vi "subVI_load_cell_KA.vi"(9 "offset":dbl, 10 "scale":dbl=1.0, 11 "DATA ARRAY IN":bool[](array[boolean])) -> (3 "LOAD OUT":dbl)   [LabVIEW 2018]
panel:
  out "decimal number":i32
  out "32 bit Zero padded array":bool[](array[boolean])
  out "24 bit Data array":bool[](array[boolean])
  # "This Sub-VI takes the Boolean Array from the Load Cell Amplifier\nand converts it into a load using the scale and offset from calibration"
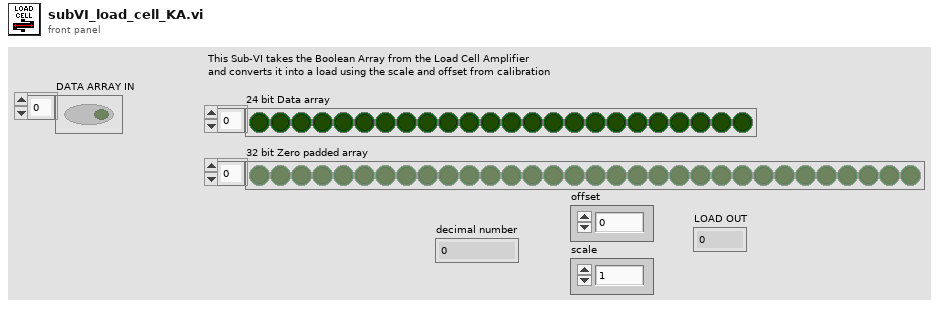
[diagram p1: front panel]
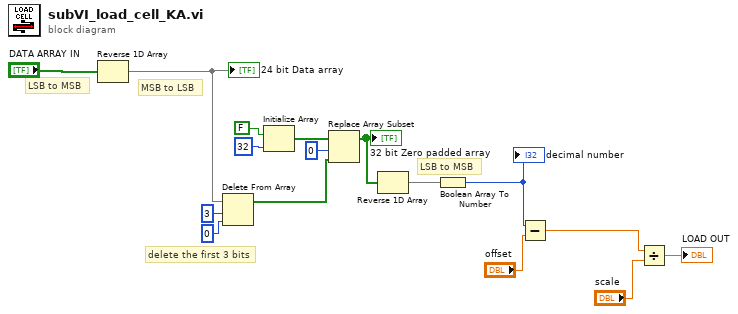
[diagram p0: block diagram]
diagram:
  # "LSB to MSB"
  # "delete the first 3 bits"
  # "LSB to MSB"
  # "MSB to LSB"
  n1 = Reverse 1D Array(array="DATA ARRAY IN") -> (reversed array=w6:bool[])
  "24 bit Data array" <- w6
  n2 = Delete From Array(array=w6, length=3, index=0) -> (array with subset deleted=w3:bool[])  [unwired: 1 out]
  n3 = Initialize Array(FALSE, 32 ("dimension size")) -> (w9:bool[])
  n4 = Replace Array Subset(array=w9, new element=w3, index=0) -> (w7:bool[])
  "32 bit Zero padded array" <- w7
  n5 = Reverse 1D Array(array=w7) -> (reversed array=w8:bool[])
  n6 = Boolean Array To Number(Boolean array=w8) -> (number=w1:i32)
  "decimal number" <- w1
  n7 = Subtract(x=w1, y="offset") -> (x-y=w14:dbl)
  n8 = Divide(x=w14, y="scale") -> (x/y=→"LOAD OUT":dbl)
